vi "Read FrameDone EvtRefNum.vi"(8 "error in (no error)":errorcluster, 11 "IMAQdx Cam in":refnum<class "IMAQdx Cam.lvclass">) -> (0 "error out":errorcluster, 2 "FrameDone":refnum<event-registration>, 3 "IMAQdx Cam out":refnum<class "IMAQdx Cam.lvclass">)   [LabVIEW 2009, in "IMAQdx Cam.lvclass"]
uses:
  IMAQdx Cam.lvclass
  IMAQdx Cam.lvclass/IMAQdx Cam.ctl
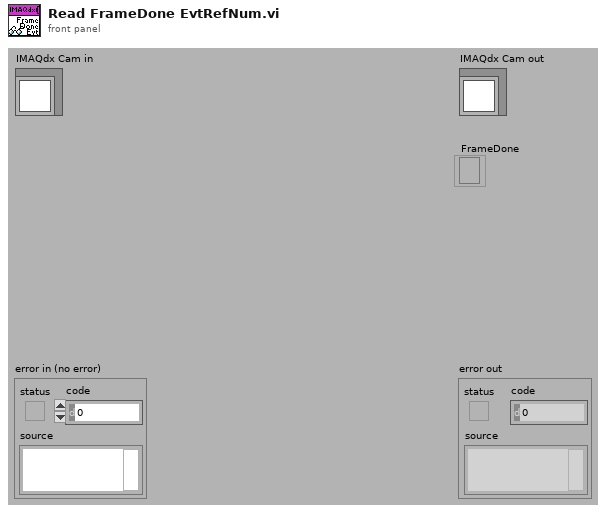
[diagram p1: front panel]
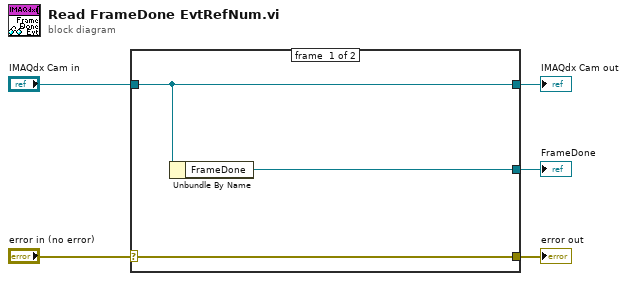
[diagram p0: block diagram]
diagram:
  n1 = case shown="No Error" "error in (no error)" {
    selector: "error in (no error)" -> [w8 w9]
    tunnel: [w8 w9] -> w4
    tunnel: [w7 w10] -> w2
    tunnel: "IMAQdx Cam in" -> [w7 w10]
    tunnel: [w6 _] -> w1
    frame #0 {
      n2 = Unbundle By Name(w7) -> ("FrameDone"=w6:refnum<event-registration>)
    }
    frame #1 {
    }
  }
  "error out" <- w4
  "IMAQdx Cam out" <- w2
  "FrameDone" <- w1
